vi "test bench_FXP_Linear_controller_observer.vi"() -> ()   [LabVIEW 2017]
uses:
  fpga_subVIs_ssxy/fixed-point-ss/typeDefs/FXPControlParams_distEst.ctl
  fpga_subVIs_ssxy/fixed-point-ss/typeDefs/UT_matrix_data.ctl
  fpga_subVIs_ssxy/fixed-point-ss/typeDefs/Bz_vec_scalar.ctl
  fpga_subVIs_ssxy/fixed-point-ss/typeDefs/Lz_vec_scalar.ctl
  fpga_subVIs_ssxy/fixed-point-ss/typeDefs/Kz_vec_scalar.ctl
  fpga_subVIs_ssxy/fixed-point-ss/typeDefs/Nx_vec_scalar.ctl
  fpga_subVIs_ssxy/fixed-point-ss/typeDefs/Az_vec_scalar.ctl
  fpga_subVIs_ssxy/fixed-point-ss/typeDefs/x_vec_scalar.ctl
  fpga_subVIs_ssxy/fixed-point-ss/typeDefs/Cz_vec_scalar.ctl
  fpga_subVIs_ssxy/fixed-point-ss/typeDefs/Kz_bram.ctl
  fpga_subVIs_ssxy/fixed-point-ss/typeDefs/A_as_vec_bram.ctl
  fpga_subVIs_ssxy/fixed-point-ss/typeDefs/Bz_bram.ctl
  fpga_subVIs_ssxy/fixed-point-ss/typeDefs/x_vec_bram.ctl
  fpga_subVIs_ssxy/fixed-point-ss/typeDefs/Lz_bram.ctl
  <vilib>/rvi/Emulation/niFpgaEmulationIsFPGAContextNoSignature.vi
  <vilib>/rvi/DataTransferAndStorage/Container/Common/niFpgaContainerGetUniqueNameForEmu.vi
  <vilib>/rvi/Memory/Memory_Emulation/niFpgaMemoryEmulationCacheClearOnFirstRun.vi
  <vilib>/rvi/Memory/Memory_Emulation/nirvimemoryEmulationManagerCache_MakeExclusive.vi
  <vilib>/rvi/Memory/Memory_Emulation/niFpgaMemoryEmulationValidateCache.vi
  <vilib>/rvi/Memory/Memory_Emulation/nirvimemoryEmulationManagerCache_InsertValue.vi
  <vilib>/Utility/error.llb/Clear Errors.vi
  <vilib>/rvi/Memory/Memory_Emulation/nirvimemoryEmulationManagerCache_ReleaseExclusive.vi
  <vilib>/rvi/Memory/Memory_Emulation/nirvimemoryEmulationManagerCache_GetValue.vi
  <vilib>/rvi/Memory/Memory_Emulation/nirvimemoryEmulationManagerCache_SetValue.vi
  <vilib>/rvi/Emulation/niFpgaProcessEmulError.vi
  <vilib>/rvi/Emulation/niFpgaSctlEmulationGetInTimedLoop.vi
  <vilib>/rvi/DataTransferAndStorage/Container/Common/niFpgaContainerExecOnDevCompGetState.vi
  <vilib>/rvi/errors/nirviReportUnexpectedCaseInternalError (U32).vi
  <vilib>/rvi/Emulation/niFpgaSctlEmulationResourceMgr.vi
  <vilib>/rvi/DataTransferAndStorage/Container/XNode/niFpgaContainer.xnode
  <vilib>/rvi/DataTransferAndStorage/Register/Emulation/niFpgaRegisterEmulation.vi
  <vilib>/rvi/Memory/Memory_Emulation/niFpgaMemoryEmulationRefIn.vi
panel:
  in  "matrix_data":T1
  in  "d_hat":fxp<+/-,32,6>
  in  "xk_1_0":fxp<+/-,32,5>[](array[numeric])=[0.0, 0.0, 0.0, 0.0, 0.0, 0.0, 0.0, 0.0, 0.0, 0.0, 0.0, 0.0, 0.0, 0.0, 0.0, 0.0, 0.0, 0.0, 0.0, 0.0, 0.0, 0.0, 0.0, 0.0, 0.0, 0.0, 0.0, 0.0, 0.0, 0.0, 0.0, 0.0, 0.0, 0.0, 0.0, 0.0, 0.0, 0.0, 0.0, 0.0, 0.0, 0.0, 0.0, 0.0, 0.0, 0.0, 0.0, 0.0, 0.0, 0.0]
  out "A*xk(out)":fxp<+/-,32,5>[](array[numeric])
  out "xk_0_1":fxp<+/-,32,5>[](array[numeric])
  out "xk_0_2":fxp<+/-,32,5>[](array[numeric])
  out "yd_est":fxp<+/-,32,5>
  in  "y(k-1)":fxp<+/-,32,5>
  in  "x_u(k)":fxp<+/-,32,8>
  out "del u(k)":fxp<+/-,64,15>
  out "u_k (saturated)":fxp<+/-,32,5>
  in  "ControlParams_distEst":T9={"umax"=3.0, "Ns_obs/cntrl"=0, "ref_f_VEC"=[0.0, 0.0], "du_max"=0.0, "Nbar"=0.0}
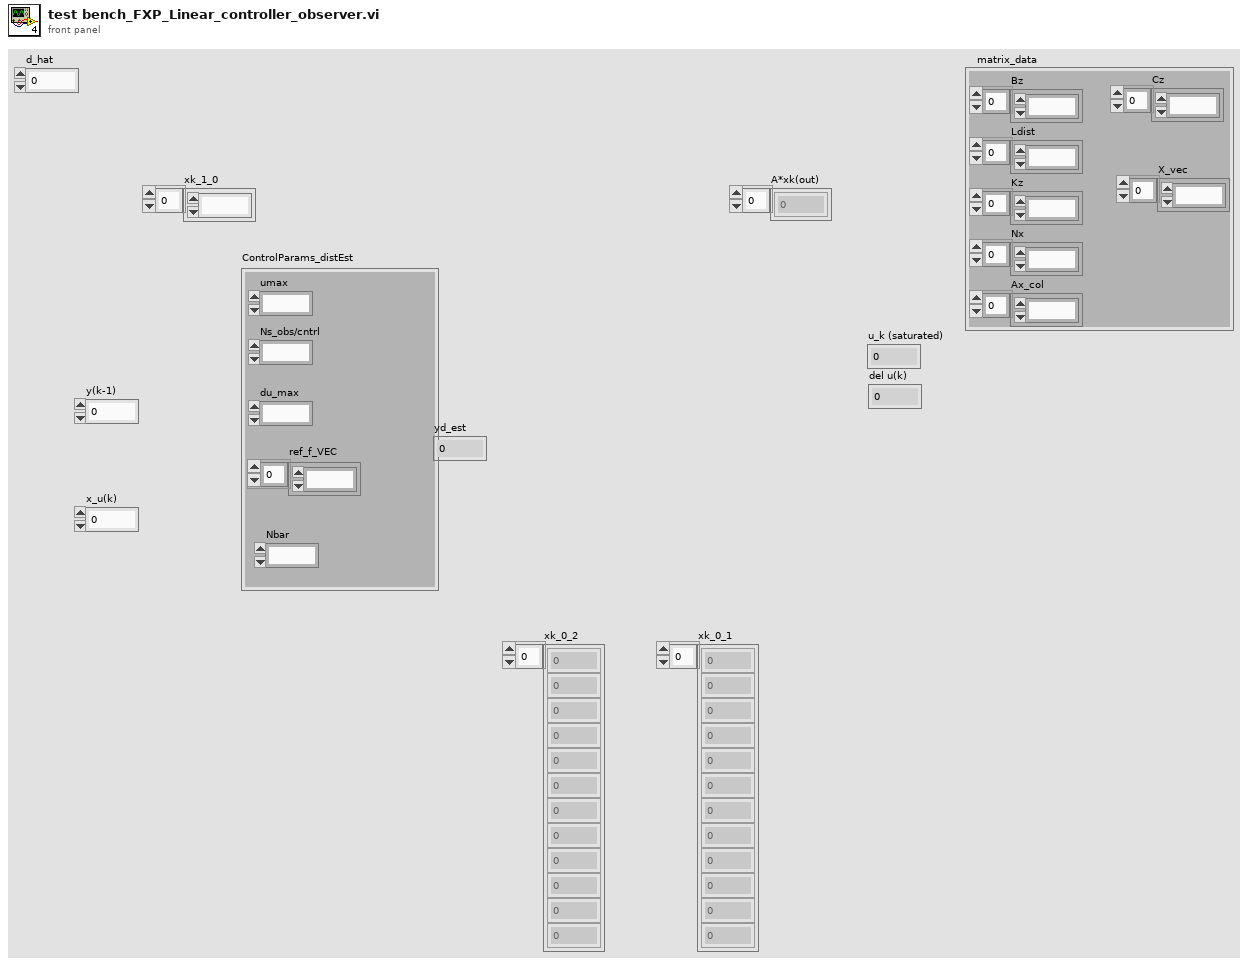
[diagram p1: front panel]
types:
  T1 = typedef "UT_matrix_data.ctl" = cluster{"Bz":T2[], "Ldist":T3[], "Kz":T4[], "Nx":T5[], "Ax_col":T6[], "X_vec":T7[], "Cz":T8[]}
  T2 = typedef "Bz_vec_scalar.ctl" = fxp<+/-,32,3>
  T3 = typedef "Lz_vec_scalar.ctl" = fxp<+/-,32,3>
  T4 = typedef "Kz_vec_scalar.ctl" = fxp<+/-,32,10>
  T5 = typedef "Nx_vec_scalar.ctl" = fxp<+/-,32,2>
  T6 = typedef "Az_vec_scalar.ctl" = fxp<+/-,32,7>
  T7 = typedef "x_vec_scalar.ctl" = fxp<+/-,32,6>
  T8 = typedef "Cz_vec_scalar.ctl" = fxp<+/-,32,4>
  T9 = typedef "FXPControlParams_distEst.ctl" = cluster{"umax":fxp<+/-,18,5>, "Ns_obs/cntrl":u8, "ref_f_VEC":fxp<+/-,32,5>[], "du_max":fxp<+/-,18,5>, "Nbar":fxp<+/-,32,5>}
  T10 = typedef "Kz_bram.ctl" = refnum<k21>
  T11 = typedef "A_as_vec_bram.ctl" = refnum<k21>
  T12 = typedef "x_vec_bram.ctl" = refnum<k21>
  T13 = typedef "Bz_bram.ctl" = refnum<k21>
  T14 = typedef "Lz_bram.ctl" = refnum<k21>
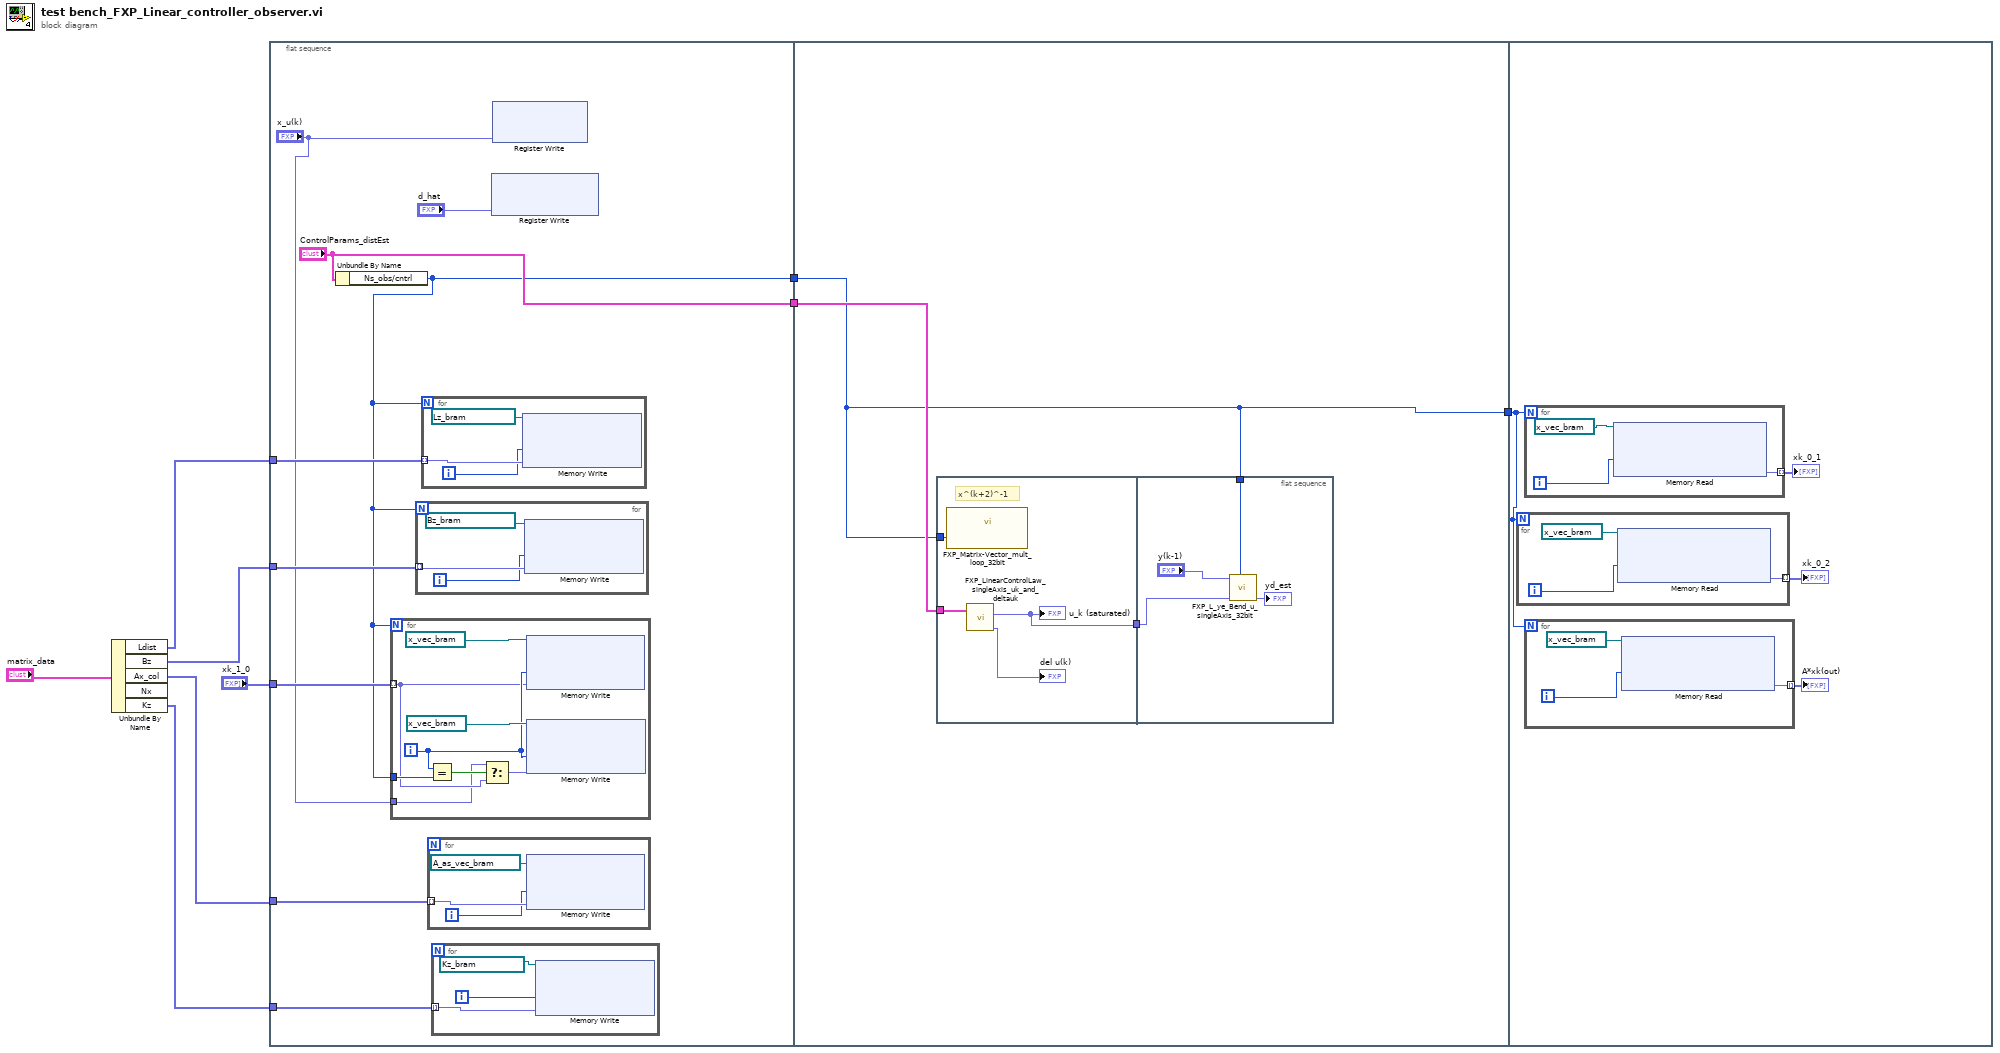
[diagram p0: block diagram]
diagram:
  n1 = Unbundle By Name("matrix_data") -> ("Ldist"=w4:T3[], "Bz"=w3:T2[], "Ax_col"=w5:T6[], "Kz"=w2:T4[])  [unwired: 1 out]
  n2 = flat-sequence {
    tunnel: w4 -> [w18]
    tunnel: "xk_1_0" -> [w17]
    tunnel: w3 -> [w16]
    tunnel: ["ControlParams_distEst"] -> w8
    tunnel: [w11] -> w7
    tunnel: w5 -> [w14]
    tunnel: w2 -> [w13]
    tunnel: [w40] -> w9
    tunnel: w8 -> [w41]
    tunnel: w7 -> [w40]
    tunnel: w9 -> [w50]
    frame #0 {
      n3 = Unbundle By Name("ControlParams_distEst") -> ("Ns_obs/cntrl"=w11:u8)
      n4 = for {
        N: w11 -> [_]
        tunnel: w17 -> [w26] mode=indexing
        tunnel: w11 -> [w30]
        tunnel: "x_u(k)" -> [w25]
        i -> [w29]
        n5 = Equal?(x=w29, y=w30) -> (x = y?=w28:bool)
        n6 = Select(t=w25, s=w28, f=w26) -> (s? t:f=w27:fxp<+/-,35,8>)
        n7 = xnode "Memory Write"("Address"=w29, "Data"=w26, "Memory In"=T12 "xk_0_1" ("Memory")) -> ()  [unwired: 1 out]
        n8 = xnode "Memory Write"("Address"=w29, "Data"=w27, "Memory In"=T12 "xk_0_2" ("Memory")) -> ()  [unwired: 1 out]
      }
      n9 = for {
        N: w11 -> [_]
        tunnel: w16 -> [w35] mode=indexing
        i -> [w34]
        n10 = xnode "Memory Write"("Address"=w34, "Data"=w35, "Memory In"=T13 "Bz_FXP_col1" ("Memory")) -> ()  [unwired: 1 out]
      }
      n11 = for {
        N: w11 -> [_]
        tunnel: w18 -> [w38] mode=indexing
        i -> [w37]
        n12 = xnode "Memory Write"("Address"=w37, "Data"=w38, "Memory In"=T14 "L_FXP_col1" ("Memory")) -> ()  [unwired: 1 out]
      }
      n13 = for {
        tunnel: w14 -> [w24] mode=indexing
        i -> [w23]
        n14 = xnode "Memory Write"("Address"=w23, "Data"=w24, "Memory In"=T11 "AasCol _FXP") -> ()  [unwired: 1 out]
      }
      n15 = for {
        tunnel: w13 -> [w21] mode=indexing
        i -> [w20]
        n16 = xnode "Memory Write"("Address"=w20, "Data"=w21, "Memory In"=T10 "K_FXP_row1" ("Memory")) -> ()  [unwired: 1 out]
      }
      n17 = xnode "Register Write"("Data"="d_hat") -> ()  [unwired: 1 in, 1 out]
      n18 = xnode "Register Write"("Data"="x_u(k)") -> ()  [unwired: 1 in, 1 out]
    }
    frame #1 {
      n19 = flat-sequence {
        tunnel: w40 -> [w44]
        tunnel: w41 -> [w43]
        tunnel: [w42] -> w39
        tunnel: w40 -> [w47]
        tunnel: w39 -> [w46]
        frame #0 {
          # "x^(k+2)^-1"
          n20 = call "FXP_Matrix-Vector_mult_loop_32bit.vi"("Ns_1"=w44) -> ()  [unwired: 10 in, 1 out]
          n21 = call "FXP_LinearControlLaw_singleAxis_uk_and_deltauk.vi"("ControlParams_distEst"=w43) -> ("del u_x"=→"del u(k)":fxp<+/-,64,15>, "u_k (un saturated)"=w42:fxp<+/-,32,5>)  [unwired: 9 in]
          "u_k (saturated)" <- w42
        }
        frame #1 {
          n22 = call "FXP_L_ye_Bend_u_singleAxis_32bit.vi"("NS"=w47, "U(k): ux"=w46, "Y(k): x"="y(k-1)") -> ("yd_est"=→"yd_est":fxp<+/-,32,5>)  [unwired: 7 in, 1 out]
        }
      }
    }
    frame #2 {
      n23 = for {
        N: w50 -> [_]
        tunnel: [w58] -> w52 mode=indexing
        i -> [w59]
        n24 = xnode "Memory Read"("Address"=w59, "Memory In"=T12 "xk_0_2" ("Memory")) -> ("Data"=w58:fxp<+/-,32,6>)  [unwired: 1 out]
      }
      "xk_0_2" <- w52
      n25 = for {
        N: w50 -> [_]
        tunnel: [w61] -> w53 mode=indexing
        i -> [w62]
        n26 = xnode "Memory Read"("Address"=w62, "Memory In"=T12 "xk_0_1" ("Memory")) -> ("Data"=w61:fxp<+/-,32,6>)  [unwired: 1 out]
      }
      "xk_0_1" <- w53
      n27 = for {
        N: w50 -> [_]
        tunnel: [w55] -> w51 mode=indexing
        i -> [w56]
        n28 = xnode "Memory Read"("Address"=w56, "Memory In"=T12 "xk_1_0" ("Memory")) -> ("Data"=w55:fxp<+/-,32,6>)  [unwired: 1 out]
      }
      "A*xk(out)" <- w51
    }
  }
